vi "USB serial.vi"() -> ()   [LabVIEW 2018]
uses:
  <vilib>/Instr/_visa.llb/VISA Configure Serial Port (Instr).vi
panel:
  out "Milliseconds":dbl format="%.3f"
  in  "MilliSeconsds":dbl(knob) scale=0.0..35.0
  in  "write buffer":string
  out "Serial Settings:Number of Bytes at Serial Port":u32
  out "error out":errorcluster
  in  "stop":bool
  out "read buffer":string
  in  "error in (no error)":errorcluster
  in  "VISA resource name":refnum<visa-resource-name>
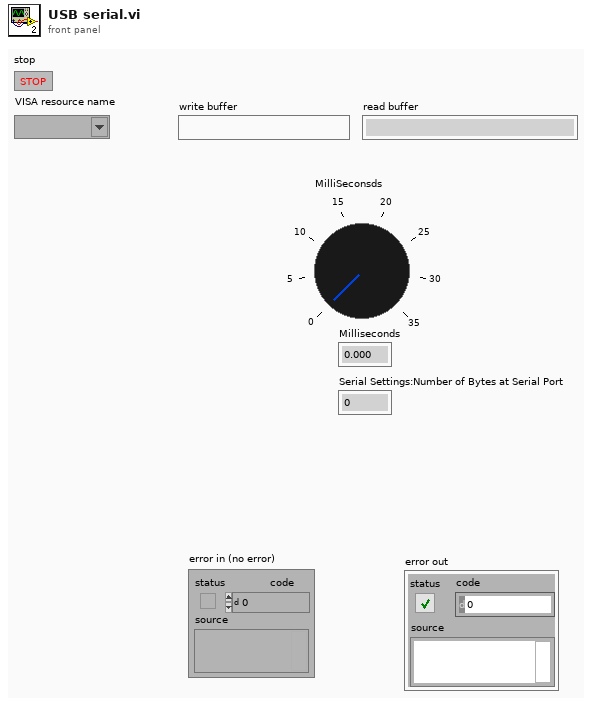
[diagram p1: front panel]
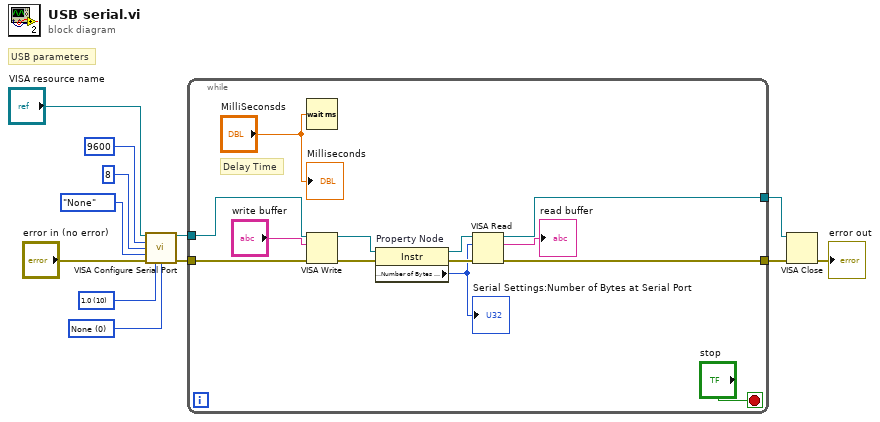
[diagram p0: block diagram]
diagram:
  w4 = u16 0 items=["None", "XON/XOFF", "RTS/CTS", "XON/XOFF & RTS/CTS", "DTR/DSR", "XON/XOFF & DTR/DSR"] ("flow control (0:none)")
  w5 = u16 10 items=["1.0"=10, "1.5"=15, "2.0"=20] ("stop bits (10: 1 bit)")
  # "USB parameters"
  n1 = call-poly "VISA Configure Serial Port"("VISA resource name"="VISA resource name", "baud rate (9600)"=u32 9600, "data bits (8)"=u16 8, "parity (0:none)"=enum16{"None", "Odd", "Even", "Mark", "Space"}."None", "error in (no error)"="error in (no error)", "stop bits (10: 1 bit)"=w5, "flow control (0:none)"=w4) -> ("VISA resource name out"=w6:refnum<visa-resource-name>, "error out"=w7:errorcluster)  [unwired: 7 in]
  n2 = while {
    tunnel: w7 -> [w25]
    tunnel: w6 -> [w24]
    tunnel: [w14] -> w3
    tunnel: [w13] -> w2
    stop <- "stop" stop-if-true
    # "Delay Time"
    n3 = Wait (ms)(milliseconds to wait="MilliSeconsds") -> ()  [unwired: 1 out]
    n4 = VISA Write(VISA resource name=w24, write buffer="write buffer", error in (no error)=w25) -> (VISA resource name out=w23:refnum<visa-resource-name>, error out=w22:errorcluster)  [unwired: 1 out]
    n5 = property on="Property Node" class="Instr"(reference=w23, error in=w22) -> (reference out=w20:refnum<visa-resource-name>, error out=w21:errorcluster, "Serial Settings:Number of Bytes at Serial Port"=w18:u32)
    "Serial Settings:Number of Bytes at Serial Port" <- w18
    n6 = VISA Read(VISA resource name=w20, byte count=w18, error in (no error)=w21) -> (VISA resource name out=w14:refnum<visa-resource-name>, read buffer=→"read buffer":string, error out=w13:errorcluster)  [unwired: 1 out]
    "Milliseconds" <- "MilliSeconsds"
  }
  n7 = VISA Close(VISA resource name=w3, error in (no error)=w2) -> (error out=→"error out":errorcluster)
